vi "LvJDS2900_Sub_SendAndRecv.vi"(8 "error in (no error)":errorcluster caption="エラー入力（エラーなし）", 10 "Command":string, 11 "VISA rsrc":refnum<visa-resource-name>) -> (0 "error out":errorcluster caption="エラー出力", 1 "Response":string, 3 "VISA rsrc out":refnum<visa-resource-name>)   [LabVIEW 2014]
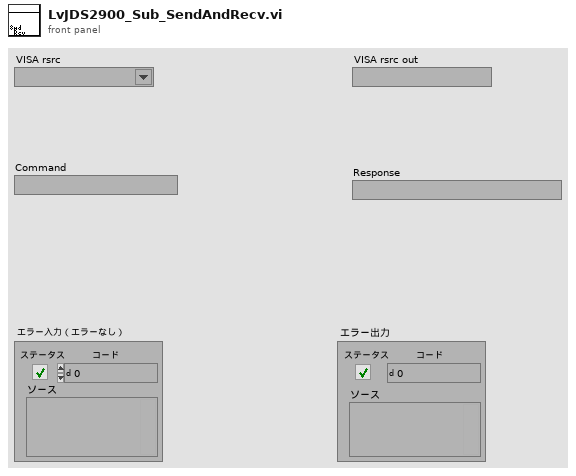
[diagram p1: front panel]
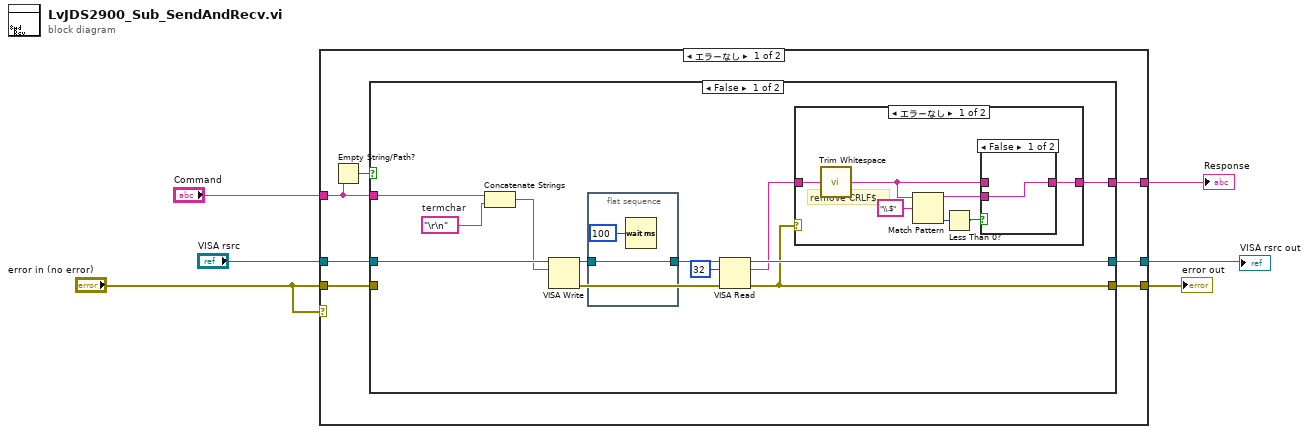
[diagram p0: block diagram]
diagram:
  n1 = case shown="エラーなし" "error in (no error)" {
    tunnel: "VISA rsrc" -> [w13 w39]
    tunnel: "Command" -> [w8 _]
    tunnel: [w12 w40] -> w4
    tunnel: "error in (no error)" -> [w11 w40]
    tunnel: [w10 w39] -> w3
    tunnel: [w9 _] -> w1
    frame No Error {
      n2 = Empty String/Path?(string/path=w8) -> (empty?=w7:bool)
      n3 = case shown="FALSE" w7 {
        tunnel: w13 -> [w25 w38]
        tunnel: w8 -> [w24 _]
        tunnel: [w16 w37] -> w12
        tunnel: w11 -> [_ w37]
        tunnel: [w21 w38] -> w10
        tunnel: [w17 _] -> w9
        frame False {
          w23 = "\r\n"  # termchar
          n4 = Concatenate Strings(w24, w23) -> (w20:string)
          n5 = VISA Write(VISA resource name=w25, write buffer=w20) -> (VISA resource name out=w15:refnum<visa-resource-name>, error out=w19:errorcluster)  [unwired: 1 in, 1 out]
          n6 = flat-sequence {
            tunnel: w15 -> [w27]
            tunnel: [w27] -> w14
            frame #0 {
              n7 = Wait (ms)(milliseconds to wait=u32 100 ("ミリ秒待機時間")) -> ()  [unwired: 1 out]
            }
          }
          n8 = VISA Read(VISA resource name=w14, byte count=u32 32 ("バイトカウント"), error in (no error)=w19) -> (VISA resource name out=w21:refnum<visa-resource-name>, read buffer=w18:string, error out=w16:errorcluster)  [unwired: 1 out]
          n9 = case shown="エラーなし" w16 {
            tunnel: w18 -> [w34 _]
            tunnel: [w29 _] -> w17
            frame No Error {
              # "remove CRLF$"
              n10 = call <vilib>:"Trim Whitespace.vi"("string"=w34) -> ("trimmed string"=w30:string)  [unwired: 1 in]
              n11 = Match Pattern(string=w30, regular expression="\\.$" ("正規表現")) -> (before substring=w28:string, offset past match=w32:i32)  [unwired: 1 in, 2 out]
              n12 = Less Than 0?(x=w32) -> (x < 0?=w31:bool)
              n13 = case shown="FALSE" w31 {
                tunnel: w30 -> [_ w36]
                tunnel: [w35 w36] -> w29
                tunnel: w28 -> [w35 _]
                frame False {
                }
                frame True {
                }
              }
            }
            frame Error {
            }
          }
        }
        frame True {
        }
      }
    }
    frame Error {
    }
  }
  "error out" <- w4
  "VISA rsrc out" <- w3
  "Response" <- w1
